vi "5-lorentzian-heat-response -- analytic derivatives -- grad and curvature -- V6.vi"(7 "action":T2=enum."onlygrads", 8 "parameters map  IN":map{T1, dbl}(c390), 10 "ω (rad/sec)":dbl=0.1 format="%#_10f") -> (0 "parameters map  OUT":map{T1, dbl}(c390), 1 "λdζ(ω)/dλ OUT":map{T1, cdb}(c390), 2 "ω out (rad/sec)":dbl=0.1 format="%#_10f", 3 "ζ(ω) OUT":cdb=0.1+0.0i format="%#_10f")   [LabVIEW 2021]
uses:
  3-lorentzian-heat-response action.ctl
  3-lorentzian-parameters.ctl
panel:
  in  "κ0":dbl(slide)=6.091279771876994e-09 min=0.0 max=0.3 step=1e-12 scale=1e-10..1e-06 scale format="%#_3p"
  in  "ζ":dbl(slide)=0.016395386176563286 min=0.0 max=0.3 step=1e-06 scale=1e-05..1000.0 scale format="%#_3p"
  in  "τN":dbl(slide)=0.0007964886373917906 min=0.0 max=0.3 step=1e-06 scale=1e-06..10.0 scale format="%#_3p"
  in  "T1":dbl(slide)=0.017784241145719432 min=0.0 max=0.3 step=1e-06 scale=0.0001..10.0 scale format="%#_3p"
  in  "τC":dbl(slide)=0.0055481925503790405 min=0.0 max=0.3 step=1e-06 scale=0.0001..10.0 scale format="%#_3p"
  in  "τS":dbl(slide)=0.01833817297436167 min=0.0 max=0.3 step=1e-06 scale=0.0001..10.0 scale format="%#_3p"
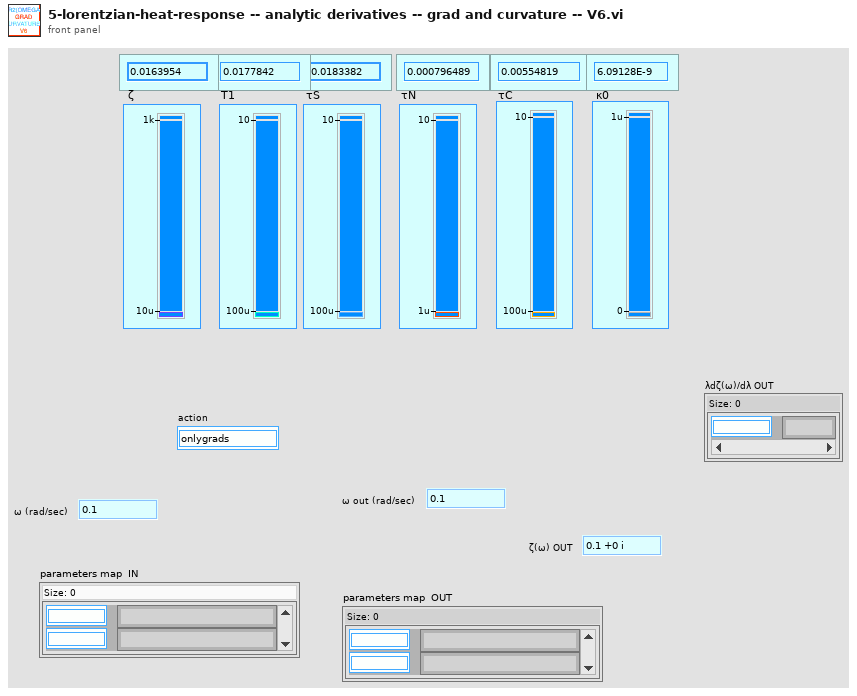
[diagram p1: front panel]
types:
  T1 = typedef "3-lorentzian-parameters.ctl" = enum16{"ζ", "τ1", "τS", "τN", "τC", "κ0", "m1", "m2", "m3", "T (K)", "B (T)", "θ (deg)", "side (S|R)", "set of (B|T)", "Re(offset)", "Im(offset)", "στ1", "στ1-", "στ1+", "στS", "στS-", "στS+", "στN", "στN-", "στN+", "τ11", "τ12", "τ21", "τ22", "τN1", "τN2"}
  T2 = typedef "3-lorentzian-heat-response action.ctl" = enum16{"calc R", "create string", "calc m1m2m3", "dζ", "dT1", "dτS", "dτN", "dτC", "d-all", "dκ0", "T(K)", "m1", "m2", "m3", "parse string", "θ (deg)", "B (T)", "onlygrads", "newton", "create emty string", "simple2nd", "calc R2", "ScalarProd", "ScalarProd-diff", "nothing", "ScalarProd-eta", "tolog", "ignore", "three2nd", "eta-errors"}
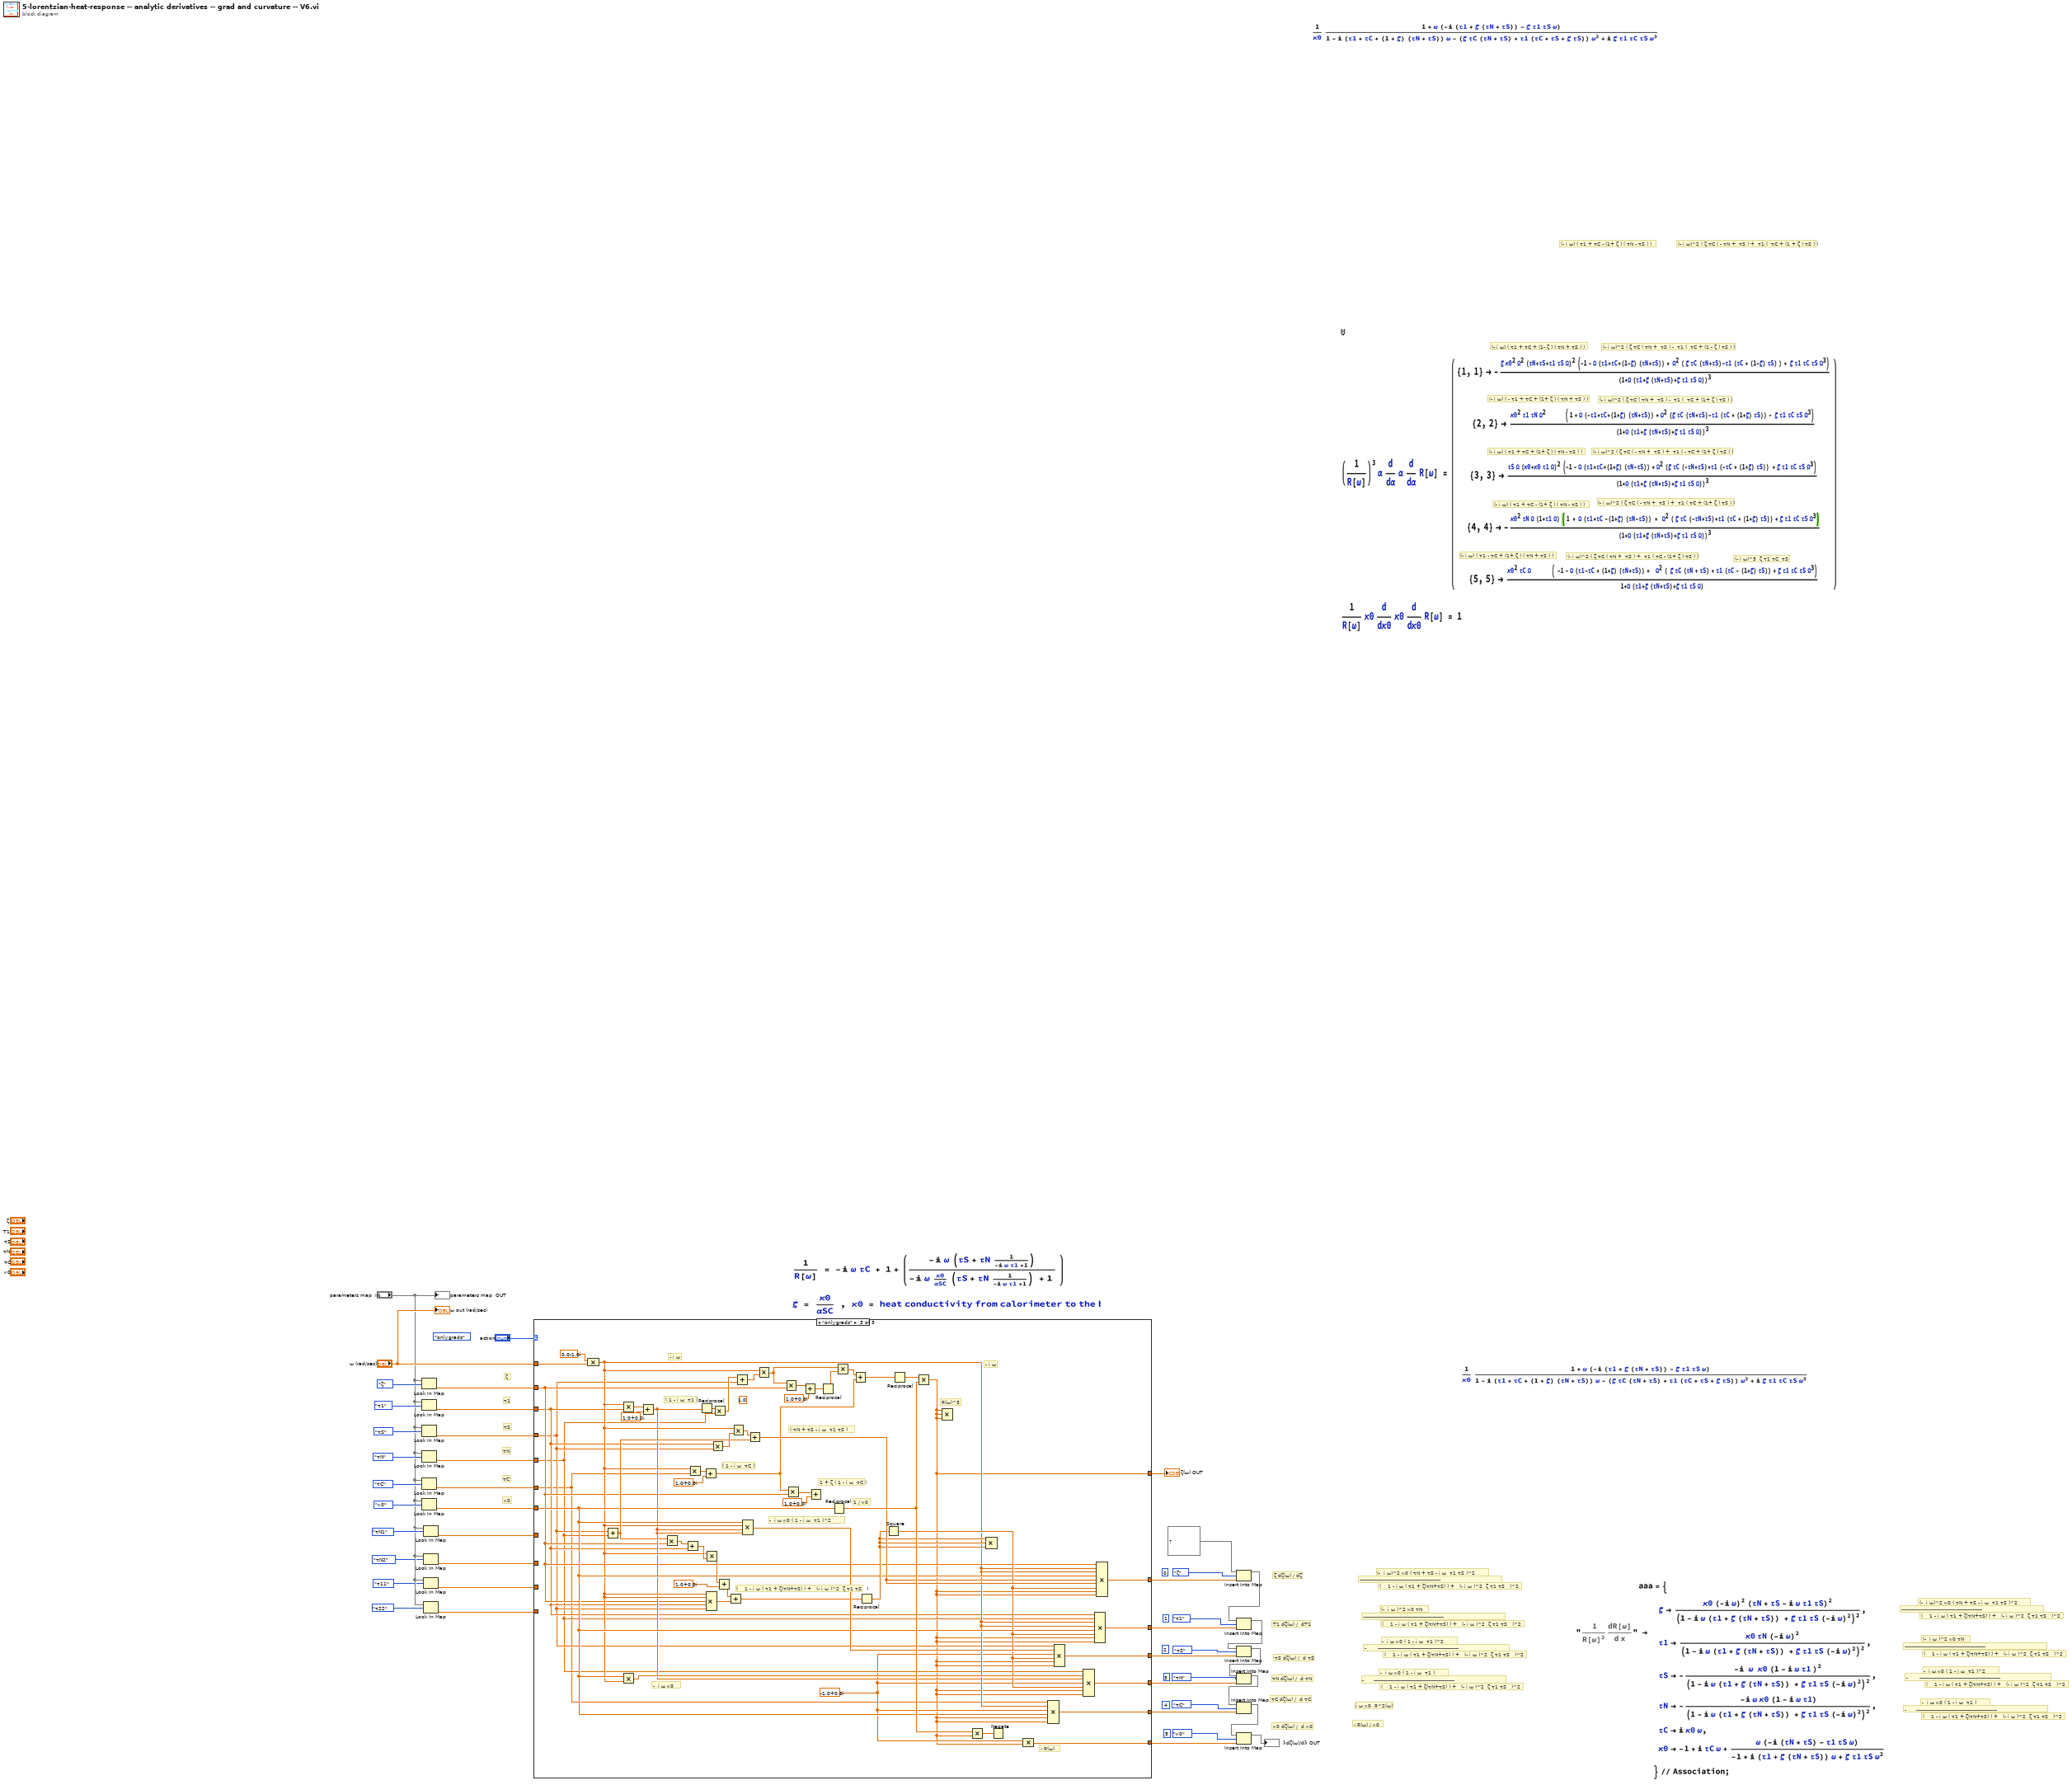
[diagram p0: block diagram]
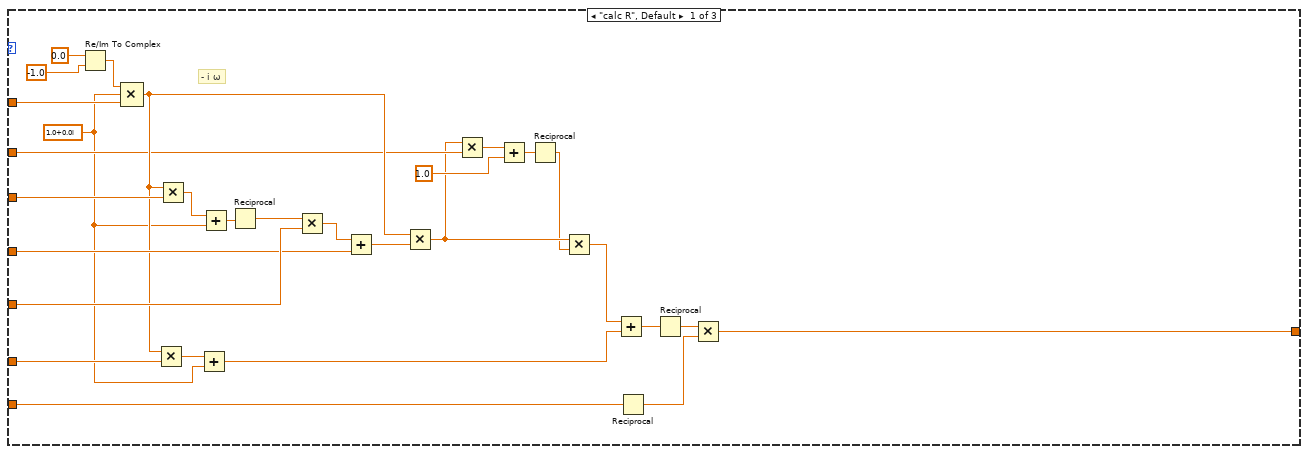
[diagram p2: hidden frame]
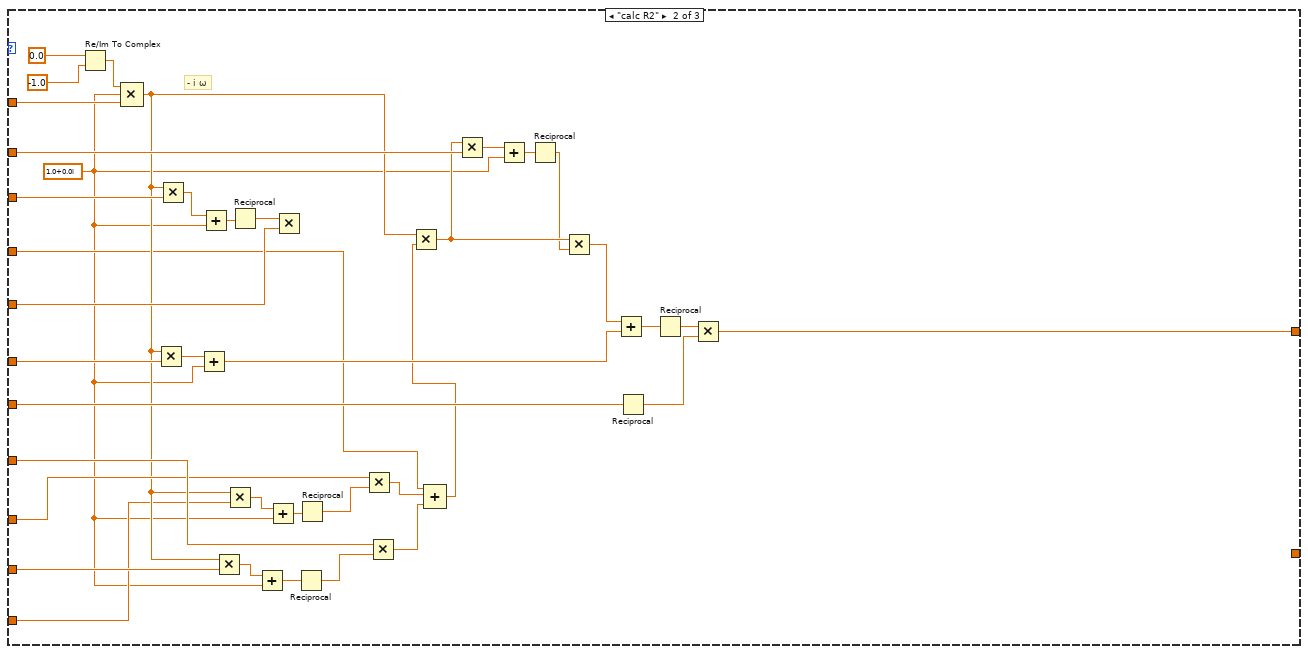
[diagram p3: hidden frame]
diagram:
  (unwired) 3-lorentzian-heat-response_action."onlygrads" ("action")
  (unwired) 5 ("key")
  (unwired) 4 ("key")
  (unwired) 3 ("key")
  (unwired) 2 ("key")
  (unwired) 1 ("key")
  (unwired) 0 ("key")
  # "κ0 dζ(ω) /  d κ0"
  # "τC dζ(ω) /  d τC"
  # "τN dζ(ω) /  d τN"
  # "τS dζ(ω) /  d τS"
  # "T1 dζ(ω) /  dT1"
  # "ζ dζ(ω) / dζ"
  # "(- i ω)^2 ( ζ τC ( - τN +  τS ) +  τ1 (  τC + (1 + ζ ) τS ) )"
  # "(- i ω) ( τ1 + τC - (1+ ζ ) ( τN - τS ) )"
  # "(- i ω)^2 ( ζ τC ( τN +  τS ) -  τ1 (  τC + (1 - ζ ) τS ) )"
  # "(- i ω) ( τ1 + τC + (1- ζ ) ( τN + τS ) )"
  # "(- i ω)^2 ( ζ τC ( τN +  τS ) -  τ1 (  τC + (1+ ζ ) τS ) )"
  # "(- i ω) ( - τ1 + τC + (1+ ζ ) ( τN + τS ) )"
  # "(- i ω)^2 ( ζ τC ( - τN +  τS ) +  τ1 ( - τC + (1+ ζ ) τS ) )"
  # "(- i ω) ( τ1 + τC + (1+ ζ ) ( τN - τS ) )"
  # "(- i ω)^2 ( ζ τC ( - τN +  τS ) +  τ1 ( τC + (1+ ζ ) τS ) )"
  # "(- i ω) ( τ1 + τC - (1+ ζ ) ( τN - τS ) )"
  # "(- i ω)^3  ζ τ1 τC  τS"
  # "(- i ω) ( τ1 - τC + (1+ ζ ) ( τN + τS ) )"
  # "(- i ω)^2 ( ζ τC ( τN +  τS ) +  τ1 ( τC - (1+ ζ ) τS ) )"
  # "κ0"
  # "τC"
  # "τN"
  # "τS"
  # "τ1"
  # "ζ"
  # "-------------------------------------------------"
  # "(-  i ω)^2 κ0 ( τN + τS - i ω  τ1 τS )^2"
  # "(    1 - i ω ( τ1 + ζ(τN+τS) ) +   (- i ω )^2  ζ τ1 τS   )^2"
  # "-------------------------------------------------"
  # "(-  i ω )^2 κ0 τN"
  # "(    1 - i ω ( τ1 + ζ(τN+τS) ) +   (- i ω )^2  ζ τ1 τS   )^2"
  # "-      -------------------------------------------------"
  # "-  i ω κ0 ( 1 - i ω  τ1 )"
  # "(    1 - i ω ( τ1 + ζ(τN+τS) ) +   (- i ω )^2  ζ τ1 τS   )^2"
  # "-       -------------------------------------------------"
  # "-  i ω κ0 ( 1 - i ω  τ1 )^2"
  # "(    1 - i ω ( τ1 + ζ(τN+τS) ) +   (- i ω )^2  ζ τ1 τS   )^2"
  # "-------------------------------------------------"
  # "(-  i ω)^2 κ0 ( τN + τS - i ω  τ1 τS )^2"
  # "(    1 - i ω ( τ1 + ζ(τN+τS) ) +   (- i ω )^2  ζ τ1 τS   )^2"
  # "-------------------------------------------------"
  # "(-  i ω )^2 κ0 τN"
  # "(    1 - i ω ( τ1 + ζ(τN+τS) ) +   (- i ω )^2  ζ τ1 τS   )^2"
  # "-      -------------------------------------------------"
  # "-  i ω κ0 ( 1 - i ω  τ1 )"
  # "(    1 - i ω ( τ1 + ζ(τN+τS) ) +   (- i ω )^2  ζ τ1 τS   )^2"
  # "-       -------------------------------------------------"
  # "-  i ω κ0 ( 1 - i ω  τ1 )^2"
  # "(    1 - i ω ( τ1 + ζ(τN+τS) ) +   (- i ω )^2  ζ τ1 τS   )^2"
  # "i ω κ0  R^2(ω)"
  # "- R(ω) / κ0"
  n1 = Look In Map(map="parameters map  IN", key=3-lorentzian-parameters."ζ" ("Plost: sweep window")) -> (value=w35:dbl)  [unwired: 1 in, 1 out]
  n2 = Look In Map(map="parameters map  IN", key=3-lorentzian-parameters."τ1" ("Plost: sweep window")) -> (value=w34:dbl)  [unwired: 1 in, 1 out]
  n3 = Look In Map(map="parameters map  IN", key=3-lorentzian-parameters."τS" ("Plost: sweep window")) -> (value=w33:dbl)  [unwired: 1 in, 1 out]
  n4 = Look In Map(map="parameters map  IN", key=3-lorentzian-parameters."τN" ("Plost: sweep window")) -> (value=w32:dbl)  [unwired: 1 in, 1 out]
  n5 = Look In Map(map="parameters map  IN", key=3-lorentzian-parameters."τC" ("Plost: sweep window")) -> (value=w31:dbl)  [unwired: 1 in, 1 out]
  n6 = Look In Map(map="parameters map  IN", key=3-lorentzian-parameters."κ0" ("Plost: sweep window")) -> (value=w30:dbl)  [unwired: 1 in, 1 out]
  n7 = Look In Map(map="parameters map  IN", key=3-lorentzian-parameters."τN1" ("Plost: sweep window")) -> (value=w3:dbl)  [unwired: 1 in, 1 out]
  n8 = Look In Map(map="parameters map  IN", key=3-lorentzian-parameters."τN2" ("Plost: sweep window")) -> (value=w2:dbl)  [unwired: 1 in, 1 out]
  n9 = Look In Map(map="parameters map  IN", key=3-lorentzian-parameters."τ11" ("Plost: sweep window")) -> (value=w4:dbl)  [unwired: 1 in, 1 out]
  n10 = Look In Map(map="parameters map  IN", key=3-lorentzian-parameters."τ22" ("Plost: sweep window")) -> (value=w1:dbl)  [unwired: 1 in, 1 out]
  n11 = case shown="\"onlygrads\"" "action" {
    tunnel: w31 -> [w61 w102 w112]
    tunnel: "ω (rad/sec)" -> [w64 w105 w162]
    tunnel: w34 -> [w63 w104 w118]
    tunnel: w32 -> [w68 w107 w116]
    tunnel: w33 -> [w66 w75 w117]
    tunnel: w35 -> [w57 w100 w119]
    tunnel: [w45 w89 w114] -> w43
    tunnel: w30 -> [w48 w92 w122]
    tunnel: [_ _ w113] -> w20
    tunnel: [_ _ w150] -> w22
    tunnel: [_ _ w139] -> w25
    tunnel: [_ _ w137] -> w24
    tunnel: [_ _ w136] -> w27
    tunnel: [_ _ w133] -> w29
    tunnel: w4 -> [_ w86 _]
    tunnel: w3 -> [_ w85 _]
    tunnel: w2 -> [_ w80 _]
    tunnel: w1 -> [_ w78 _]
    frame "calc R", Default {
      w44 = cdb 1.0+0.0i ("value")
      # "- i ω"
      n12 = Re/Im To Complex(1:-1.0 ("y"), 2:0.0 ("x")) -> (0:w65:cdb)
      n13 = Compound Arithmetic op=MULTIPLY(w65, w44, w64) -> (w59:cdb)
      n14 = Multiply(x=w59, y=w61) -> (x*y=w60:cdb)
      n15 = Multiply(x=w59, y=w63) -> (x*y=w62:cdb)
      n16 = Add(x=w60, y=w44) -> (x+y=w51:cdb)
      n17 = Add(x=w62, y=w44) -> (x+y=w70:cdb)
      n18 = Reciprocal(x=w70) -> (1/x=w69:cdb)
      n19 = Multiply(x=w69, y=w68) -> (x*y=w67:cdb)
      n20 = Add(x=w67, y=w66) -> (x+y=w58:cdb)
      n21 = Multiply(x=w59, y=w58) -> (x*y=w53:cdb)
      n22 = Multiply(x=w53, y=w57) -> (x*y=w55:cdb)
      n23 = Add(x=w55, y=1.0) -> (x+y=w54:cdb)
      n24 = Reciprocal(x=w54) -> (1/x=w52:cdb)
      n25 = Multiply(x=w53, y=w52) -> (x*y=w50:cdb)
      n26 = Add(x=w50, y=w51) -> (x+y=w49:cdb)
      n27 = Reciprocal(x=w48) -> (1/x=w46:dbl)
      n28 = Reciprocal(x=w49) -> (1/x=w47:cdb)
      n29 = Multiply(x=w47, y=w46) -> (x*y=w45:cdb)
    }
    frame "calc R2" {
      w73 = cdb 1.0+0.0i ("value")
      # "- i ω"
      n30 = Re/Im To Complex(1:-1.0 ("y"), 2:0.0 ("x")) -> (0:w106:cdb)
      n31 = Compound Arithmetic op=MULTIPLY(w106, w73, w105) -> (w79:cdb)
      n32 = Multiply(x=w79, y=w102) -> (x*y=w101:cdb)
      n33 = Multiply(x=w79, y=w104) -> (x*y=w103:cdb)
      n34 = Add(x=w101, y=w73) -> (x+y=w95:cdb)
      n35 = Add(x=w103, y=w73) -> (x+y=w109:cdb)
      n36 = Multiply(x=w79, y=w86) -> (x*y=w87:cdb)
      n37 = Multiply(x=w79, y=w78) -> (x*y=w82:cdb)
      n38 = Reciprocal(x=w109) -> (1/x=w108:cdb)
      n39 = Add(x=w87, y=w73) -> (x+y=w88:cdb)
      n40 = Add(x=w82, y=w73) -> (x+y=w83:cdb)
      n41 = Multiply(x=w108, y=w107) -> ()  [unwired: 1 out]
      n42 = Reciprocal(x=w88) -> (1/x=w84:cdb)
      n43 = Reciprocal(x=w83) -> (1/x=w81:cdb)
      n44 = Multiply(x=w80, y=w81) -> (x*y=w76:cdb)
      n45 = Multiply(x=w85, y=w84) -> (x*y=w77:cdb)
      n46 = Compound Arithmetic op=ADD(w75, w76, w77) -> (w74:cdb)
      n47 = Multiply(x=w79, y=w74) -> (x*y=w97:cdb)
      n48 = Multiply(x=w97, y=w100) -> (x*y=w99:cdb)
      n49 = Add(x=w99, y=w73) -> (x+y=w98:cdb)
      n50 = Reciprocal(x=w98) -> (1/x=w96:cdb)
      n51 = Multiply(x=w97, y=w96) -> (x*y=w94:cdb)
      n52 = Add(x=w94, y=w95) -> (x+y=w93:cdb)
      n53 = Reciprocal(x=w92) -> (1/x=w90:dbl)
      n54 = Reciprocal(x=w93) -> (1/x=w91:cdb)
      n55 = Multiply(x=w91, y=w90) -> (x*y=w89:cdb)
    }
    frame "onlygrads" {
      w115 = cdb -1.0+0.0i ("value")
      (unwired) 1.0
      # "1 + ζ ( 1 - i ω  τC )"
      # "( 1 - i ω  τC )"
      # "R(ω)^3"
      # "( τN + τS - i ω  τ1 τS )"
      # "-  i ω κ0"
      # "( 1 - i ω  τ1 )"
      # "(    1 - i ω ( τ1 + ζ(τN+τS) ) +   (- i ω )^2  ζ τ1 τS   )"
      # "-  i ω κ0 ( 1 - i ω  τ1 )^2"
      # "- i ω"
      # "1 / κ0"
      # "- R(ω)"
      # "- i ω"
      n56 = Compound Arithmetic op=MULTIPLY(cdb 0.0-1.0i ("value"), w162) -> (w121:cdb)
      n57 = Add(x=w117, y=w116) -> (x+y=w125:dbl)
      n58 = Multiply(x=w121, y=w118) -> (x*y=w130:cdb)
      n59 = Multiply(x=w122, y=w121) -> (x*y=w138:cdb)
      n60 = Add(x=w130, y=cdb 1.0+0.0i ("value")) -> (x+y=w120:cdb)
      n61 = Multiply(x=w125, y=w119) -> (x*y=w146:dbl)
      n62 = Add(x=w146, y=w118) -> (x+y=w145:dbl)
      n63 = Multiply(x=w121, y=w112) -> (x*y=w161:cdb)
      n64 = Reciprocal(x=w120) -> (1/x=w164:cdb)
      n65 = Add(x=w161, y=cdb 1.0+0.0i ("value")) -> (x+y=w128:cdb)
      n66 = Multiply(x=w121, y=w145) -> (x*y=w144:cdb)
      n67 = Compound Arithmetic op=MULTIPLY(w121, w121, w119, w118, w117) -> (w141:cdb)
      n68 = Multiply(x=w118, y=w117) -> (x*y=w135:dbl)
      n69 = Multiply(x=w164, y=w116) -> (x*y=w163:cdb)
      n70 = Add(x=w144, y=cdb 1.0+0.0i ("value")) -> (x+y=w142:cdb)
      n71 = Add(x=w142, y=w141) -> (x+y=w131:cdb)
      n72 = Multiply(x=w121, y=w135) -> (x*y=w134:cdb)
      n73 = Add(x=w163, y=w117) -> (x+y=w160:cdb)
      n74 = Compound Arithmetic op=MULTIPLY(w122, w121, w120, w120) -> (w140:cdb)
      n75 = Add(x=w134, y=w125) -> (x+y=w129:cdb)
      n76 = Multiply(x=w121, y=w160) -> (x*y=w157:cdb)
      n77 = Multiply(x=w157, y=w119) -> (x*y=w159:cdb)
      n78 = Multiply(x=w128, y=w119) -> (x*y=w127:cdb)
      n79 = Add(x=w159, y=cdb 1.0+0.0i ("value")) -> (x+y=w158:cdb)
      n80 = Add(x=w127, y=cdb 1.0+0.0i ("value")) -> ()  [unwired: 1 out]
      n81 = Reciprocal(x=w158) -> (1/x=w156:cdb)
      n82 = Reciprocal(x=w122) -> (1/x=w152:dbl)
      n83 = Multiply(x=w157, y=w156) -> (x*y=w155:cdb)
      n84 = Add(x=w155, y=w128) -> (x+y=w154:cdb)
      n85 = Reciprocal(x=w131) -> (1/x=w124:cdb)
      n86 = Square(x=w124) -> (x^2=w123:cdb)
      n87 = Reciprocal(x=w154) -> (1/x=w153:cdb)
      n88 = Multiply(x=w153, y=w152) -> (x*y=w114:cdb)
      n89 = Compound Arithmetic op=MULTIPLY(w114, w114, w114) -> ()  [unwired: 1 out]
      n90 = Multiply(x=w152, y=w114) -> (x*y=w151:cdb)
      n91 = Compound Arithmetic op=MULTIPLY(w124, w124, w124) -> ()  [unwired: 1 out]
      n92 = Negate(x=w151) -> ()  [unwired: 1 out]
      n93 = Compound Arithmetic op=MULTIPLY(w115, w114) -> (w113:cdb)
      n94 = Compound Arithmetic op=MULTIPLY(w112, w121, w115, w122, w114, w114) -> (w150:cdb)
      n95 = Compound Arithmetic op=MULTIPLY(w117, w140, w115, w123, w114, w114) -> (w139:cdb)
      n96 = Compound Arithmetic op=MULTIPLY(w116, w138, w120, w115, w123, w114, w114) -> (w137:cdb)
      n97 = Compound Arithmetic op=MULTIPLY(w118, w116, w121, w121, w122, w123, w114, w114) -> (w136:cdb)
      n98 = Compound Arithmetic op=MULTIPLY(w119, w121, w121, w122, w129, w129, w123, w114, w114) -> (w133:cdb)
    }
  }
  "ζ(ω) OUT" <- w43
  n99 = Insert Into Map(map in=map{T1, cdb} {} ("parameters map  IN 2"), key=3-lorentzian-parameters."ζ" ("Plost: sweep window"), value=w29) -> (map out=w28:map{T1, cdb})  [unwired: 2 out]
  n100 = Insert Into Map(map in=w28, key=3-lorentzian-parameters."τ1" ("Plost: sweep window"), value=w27) -> (map out=w26:map{T1, cdb})  [unwired: 2 out]
  n101 = Insert Into Map(map in=w26, key=3-lorentzian-parameters."τS" ("Plost: sweep window"), value=w25) -> (map out=w19:map{T1, cdb})  [unwired: 2 out]
  n102 = Insert Into Map(map in=w19, key=3-lorentzian-parameters."τN" ("Plost: sweep window"), value=w24) -> (map out=w23:map{T1, cdb})  [unwired: 2 out]
  n103 = Insert Into Map(map in=w23, key=3-lorentzian-parameters."τC" ("Plost: sweep window"), value=w22) -> (map out=w21:map{T1, cdb})  [unwired: 2 out]
  n104 = Insert Into Map(map in=w21, key=3-lorentzian-parameters."κ0" ("Plost: sweep window"), value=w20) -> (map out=→"λdζ(ω)/dλ OUT":map{T1, cdb})  [unwired: 2 out]
  "ω out (rad/sec)" <- "ω (rad/sec)"
  "parameters map  OUT" <- "parameters map  IN"
